vi "HEWH RLT Write Channel Multi.vi"(8 "Error In":errorcluster, 9 "Panel 3":T1[][](array[typedef]), 10 "Panel 2":T1[][](array[typedef]), 11 "Panel 1":T1[][](array[typedef])) -> (0 "Error Out":errorcluster, 3 "Write Array Out":string[][](array[string]))   [LabVIEW 2020]
uses:
  Type Definitions/HEWH Channel Label RLT.ctl
  Custom Instrument Control/MW100/Type Definitions/Station ID Selector.ctl
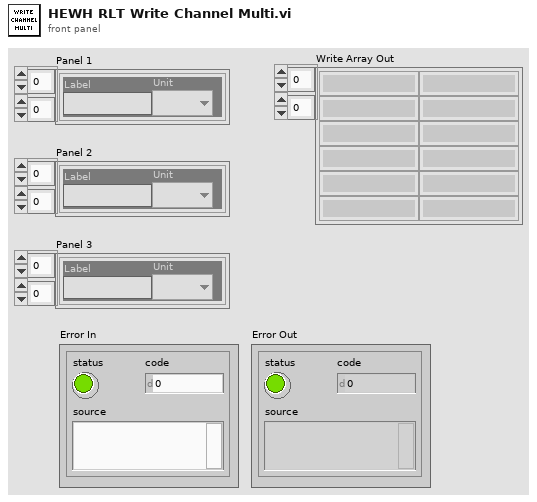
[diagram p1: front panel]
types:
  T1 = typedef "HEWH Channel Label RLT.ctl" = cluster{"Label":string, "Unit":T2}
  T2 = typedef "Station ID Selector.ctl" = enum16{"", "A", "B", "C", "D", "Global"}
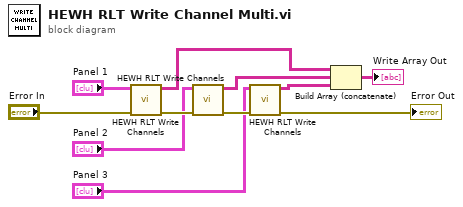
[diagram p0: block diagram]
diagram:
  n1 = call "HEWH RLT Write Channels.vi"("Error In"="Error In", "Panel Input"="Panel 1") -> ("Error Out"=w10:errorcluster, "Write Array"=w4:string[][])  [unwired: 8 in]
  n2 = call "HEWH RLT Write Channels.vi"("Error In"=w10, "Panel Input"="Panel 2") -> ("Error Out"=w11:errorcluster, "Write Array"=w7:string[][])  [unwired: 8 in]
  n3 = call "HEWH RLT Write Channels.vi"("Error In"=w11, "Panel Input"="Panel 3") -> ("Error Out"=→"Error Out":errorcluster, "Write Array"=w9:string[][])  [unwired: 8 in]
  n4 = Build Array (concatenate)(w4, w7, w9) -> (→"Write Array Out":string[][])
